vi "pockelscellzstage.vi"(0 "current slice":i32, 1 "# of Slices":u32, 4 "wavelength (nm)":dbl, 5 "Z0":dbl=50.15 caption="Z0 (start of slice)", 6 "exp?":bool, 7 "Zstart":dbl=50.15, 8 "Pend":dbl=51.15, 9 "Pstart":dbl=50.15, 10 "Z":dbl=50.15, 11 "Zend":dbl=51.15) -> (3 "T(%)":dbl)   [LabVIEW 2015]
uses:
  <vilib>/DAQmx/write.llb/DAQmx Write (Analog DBL 1Chan 1Samp).vi
  <vilib>/DAQmx/create/channels.llb/DAQmx Create Channel (AO-Voltage-Basic).vi
  <vilib>/DAQmx/miscellaneous.llb/DAQmx Fill In Error Info.vi
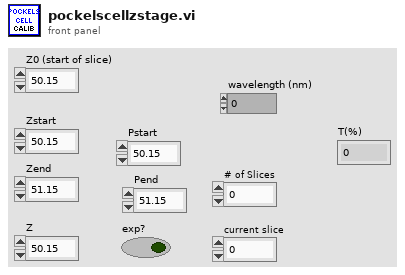
[diagram p1: front panel]
types:
  T1 = cluster{"StageS":i32, "StageL":i32, "currmeas data dir":path, "image OD":u16, "contour OD":u16, "point OD":u16, "AOlines":tag[], "AIlines":tag[], "CI lines":tag[], "DO lines":tag[], "AO names":string[], "CI names":string[], "AI names":string[], "DO names":string[], "CIextensions":string[], "AIextensions":string[], "Voltage to Ygalvo":i32, "Voltage to Xgalvo":i32, "Voltage to patch":i32, "640 shutter":i32, "2P shutter":i32, "LT timestamp":u32, "Vp":i32, "Ip":i32, "camera trigger":i32, "master data dir":path, "voltage to Zpos":i32, "Vto2P":i32, "640 AO":i32, "488 AO":i32, "532 AO":i32, "640TTL":u32, "488TTL":u32, "532TTL":u32, "Device 1 sampleclock out":tag, "Device 1 Starttrigger out":tag, "Device 2 sampleclock in":tag, "Device 2 StartTrigger in ":tag, "2PODTTL":u32, "488 shutter":u32, "LCVR red":u32, "LCVR blue":u32}
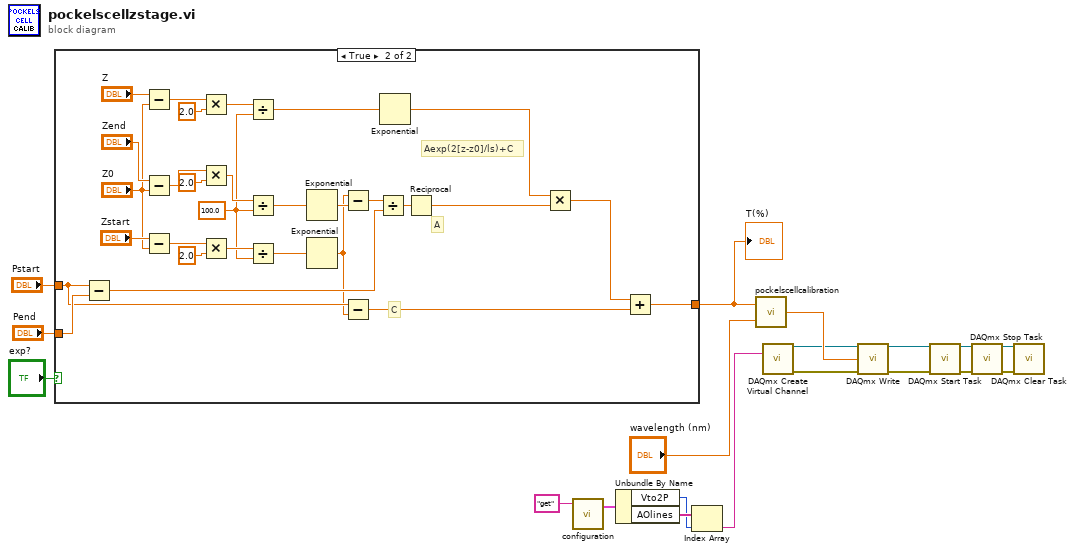
[diagram p0: block diagram]
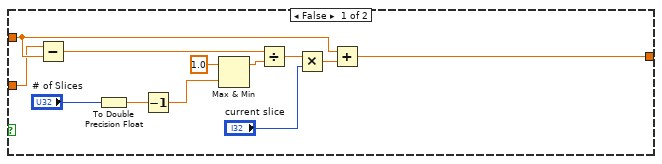
[diagram p2: hidden frame]
diagram:
  n1 = case shown="True" "exp?" {
    tunnel: "Pend" -> [w21 w52]
    tunnel: "Pstart" -> [w22 w46]
    tunnel: [w20 w33] -> w2
    frame False {
      n2 = Subtract(x=w21, y=w22) -> (x-y=w27:dbl)
      n3 = To Double Precision Float(number="# of Slices") -> (double precision float=w28:dbl)
      n4 = Decrement(x=w28) -> (x-1=w23:dbl)
      n5 = Max & Min(x=1.0 ("y"), y=w23) -> (max(x,y)=w26:dbl)  [unwired: 1 out]
      n6 = Divide(x=w27, y=w26) -> (x/y=w25:dbl)
      n7 = Multiply(x=w25, y="current slice") -> (x*y=w30:dbl)
      n8 = Add(x=w22, y=w30) -> (x+y=w20:dbl)
    }
    frame True {
      w38 = 100.0 ("Zend 2")
      # "C"
      # "A"
      # "Aexp(2[z-z0]/ls)+C"
      n9 = Subtract(x=w46, y=w52) -> (x-y=w51:dbl)
      n10 = Subtract(x="Z", y="Z0") -> (x-y=w44:dbl)
      n11 = Subtract(x="Zend", y="Z0") -> (x-y=w47:dbl)
      n12 = Subtract(x="Zstart", y="Z0") -> (x-y=w49:dbl)
      n13 = Multiply(x=w44, y=2.0) -> (x*y=w42:dbl)
      n14 = Multiply(x=w47, y=2.0) -> (x*y=w56:dbl)
      n15 = Multiply(x=w49, y=2.0) -> (x*y=w59:dbl)
      n16 = Divide(x=w42, y=w38) -> (x/y=w43:dbl)
      n17 = Divide(x=w56, y=w38) -> (x/y=w57:dbl)
      n18 = Divide(x=w59, y=w38) -> (x/y=w58:dbl)
      n19 = Exponential(1:w57) -> (0:w54:dbl)
      n20 = Exponential(1:w58) -> (0:w45:dbl)
      n21 = Subtract(x=w45, y=w54) -> (x-y=w53:dbl)
      n22 = Subtract(x=w46, y=w45) -> (x-y=w34:dbl)
      n23 = Divide(x=w53, y=w51) -> (x/y=w36:dbl)
      n24 = Exponential(1:w43) -> (0:w37:dbl)
      n25 = Reciprocal(x=w36) -> (1/x=w32:dbl)
      n26 = Multiply(x=w37, y=w32) -> (x*y=w35:dbl)
      n27 = Add(x=w35, y=w34) -> (x+y=w33:dbl)
    }
  }
  "T(%)" <- w2
  n28 = call "configuration.vi"("command"="get") -> ("config out"=w14:T1)  [unwired: 2 in, 1 out]
  n29 = Unbundle By Name(w14) -> ("Vto2P"=w15:i32, "AOlines"=w16:tag[])
  n30 = Index Array(array=w16, index=w15) -> (element=w17:tag)
  n31 = call "pockelscellcalibration.vi"("l"="wavelength (nm)", "T"=w2) -> ("Vout"=w18:dbl)
  n32 = call-poly <vilib>:"DAQmx Create Virtual Channel.vi"("physical channels"=w17) -> ("task out"=w11:refnum<k21>, "error out"=w12:errorcluster)  [unwired: 13 in]
  n33 = call-poly <vilib>:"DAQmx Write.vi"("task/channels in"=w11, "data"=w18, "error in"=w12) -> ("task out"=w10:refnum<k21>, "error out"=w9:errorcluster)  [unwired: 10 in, 1 out]
  n34 = call <vilib>:"DAQmx Start Task.vi"("task/channels in"=w10, "error in"=w9) -> ("task out"=w8:refnum<k21>, "error out"=w7:errorcluster)  [unwired: 12 in]
  n35 = call <vilib>:"DAQmx Stop Task.vi"("task/channels in"=w8, "error in"=w7) -> ("task out"=w6:refnum<k21>, "error out"=w5:errorcluster)  [unwired: 12 in]
  n36 = call <vilib>:"DAQmx Clear Task.vi"("task in"=w6, "error in"=w5) -> ()  [unwired: 13 in, 1 out]
